vi "Get Row From Double Click.vi"(8 "错误输入":errorcluster, 11 "Listbox Ref":refnum<vi>) -> (0 "错误输出":errorcluster, 2 "Get DblClk Row":i32, 3 "Dup Listbox Ref":refnum<vi>)   [LabVIEW 2012, in "Listbox Tool.lvlib"]
uses:
  Listbox Tool.lvlib
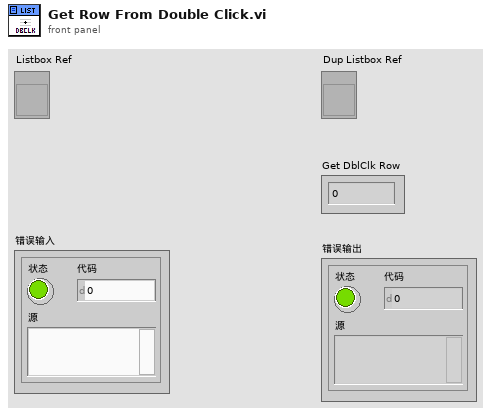
[diagram p1: front panel]
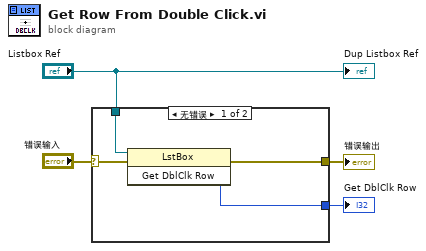
[diagram p0: block diagram]
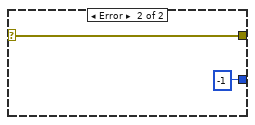
[diagram p2: hidden frame]
diagram:
  n1 = case shown="无错误" "错误输入" {
    selector: "错误输入" -> [w6 w10]
    tunnel: "Listbox Ref" -> [w8 _]
    tunnel: [w7 w10] -> w2
    tunnel: [w5 -1 ("Get DblClk Row")] -> w1
    frame No Error {
      n2 = invoke class="LstBox" method="Get DblClk Row"(reference=w8, error in=w6) -> (error out=w7:errorcluster, "Get DblClk Row"=w5:i32)  [unwired: 1 in, 1 out]
    }
    frame Error {
    }
  }
  "错误输出" <- w2
  "Get DblClk Row" <- w1
  "Dup Listbox Ref" <- "Listbox Ref"
